vi "0.SAVE_subVI.vi"(8 "1D data":dbl[](array[numeric]), 9 "2D data":dbl[][](array[numeric]), 11 "file name":string) -> ()   [LabVIEW 2020]
uses:
  <vilib>/Utility/file.llb/Write Delimited Spreadsheet (DBL).vi
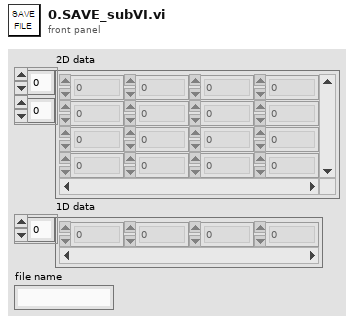
[diagram p1: front panel]
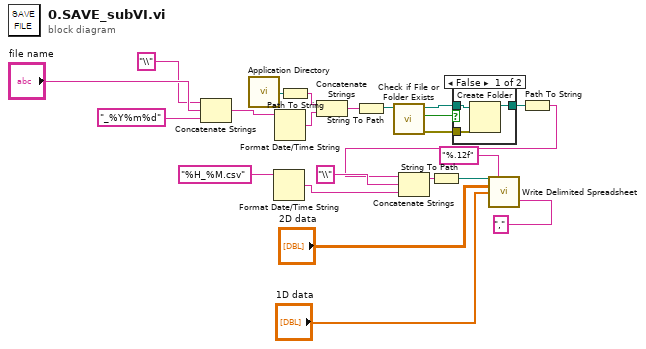
[diagram p0: block diagram]
diagram:
  n1 = Concatenate Strings("\\" ("string"), "file name", "_%Y%m%d" ("time format string (%c)")) -> (w5:string)
  n2 = call <vilib>:"Application Directory.vi"() -> ("Application Directory"=w17:path)
  n3 = Format Date/Time String(time format string (%c)="%H_%M.csv") -> (date/time string=w21:string)  [unwired: 2 in]
  n4 = Format Date/Time String(time format string (%c)=w5) -> (date/time string=w19:string)  [unwired: 2 in]
  n5 = Path To String(path=w17) -> (string=w18:string)
  n6 = Concatenate Strings(w18, w19) -> (w16:string)
  n7 = String To Path(string=w16) -> (path=w15:path)
  n8 = call <vilib>:"Check if File or Folder Exists.vi"("path"=w15) -> ("error out"=w14:errorcluster, "file or folder exists?"=w12:bool, "dup path"=w13:path)  [unwired: 8 in]
  n9 = case shown="False" w12 {
    tunnel: w13 -> [w26 w27]
    tunnel: w14 -> [w25 _]
    tunnel: [w24 w27] -> w20
    frame False {
      n10 = Create Folder(path (use dialog)=w26, error in=w25) -> (created path=w24:path)  [unwired: 1 in, 2 out]
    }
    frame True {
    }
  }
  n11 = Path To String(path=w20) -> (string=w9:string)
  n12 = Concatenate Strings(w9, "\\" ("string"), w21) -> (w22:string)
  n13 = String To Path(string=w22) -> (path=w23:path)
  n14 = call-poly <vilib>:"Write Delimited Spreadsheet.vi"("file path (dialog if empty)"=w23, "format (%.3f)"="%.12f", "2D data"="2D data", "1D data"="1D data", "delimiter (\\t)"="," ("delimiter (\\t)")) -> ()  [unwired: 9 in, 2 out]
